vi "Rep Rate To Num Samples.vi"(4 "Sampling Rate (Hz)":dbl, 5 "Rep Rate (Hz)":dbl) -> (1 "Samples/period":i32)   [LabVIEW 2015]
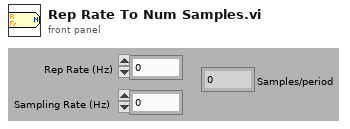
[diagram p1: front panel]
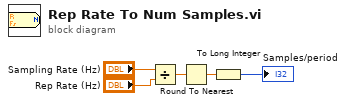
[diagram p0: block diagram]
diagram:
  n1 = Divide(x="Sampling Rate (Hz)", y="Rep Rate (Hz)") -> (x/y=w4:dbl)
  n2 = Round To Nearest(number=w4) -> (nearest integer value=w3:dbl)
  n3 = To Long Integer(number=w3) -> (32bit integer=→"Samples/period":i32)
